vi "viewer0.1.vi"() -> ()   [LabVIEW 2020]
uses:
  <vilib>/Utility/file.llb/Read Delimited Spreadsheet (DBL).vi
panel:
  out "Intensity Graph 4":i32[][](graph)
  in  "Numeric":i32
  out "f":dbl=13.10591113674956
  out "t":dbl=0.07630144822178409
  in  "file path (dialog if empty)":path=path "W:/Labview/Front ends/ARPEScontrol/testfiles/1x1"
  out "Intensity Graph":dbl[][](graph)
  in  "e-size":u8=5
  in  "square thresh":i32=50
  in  "delta thresh":dbl=1.0
  in  "subtract":dbl=10.0
  # "4"
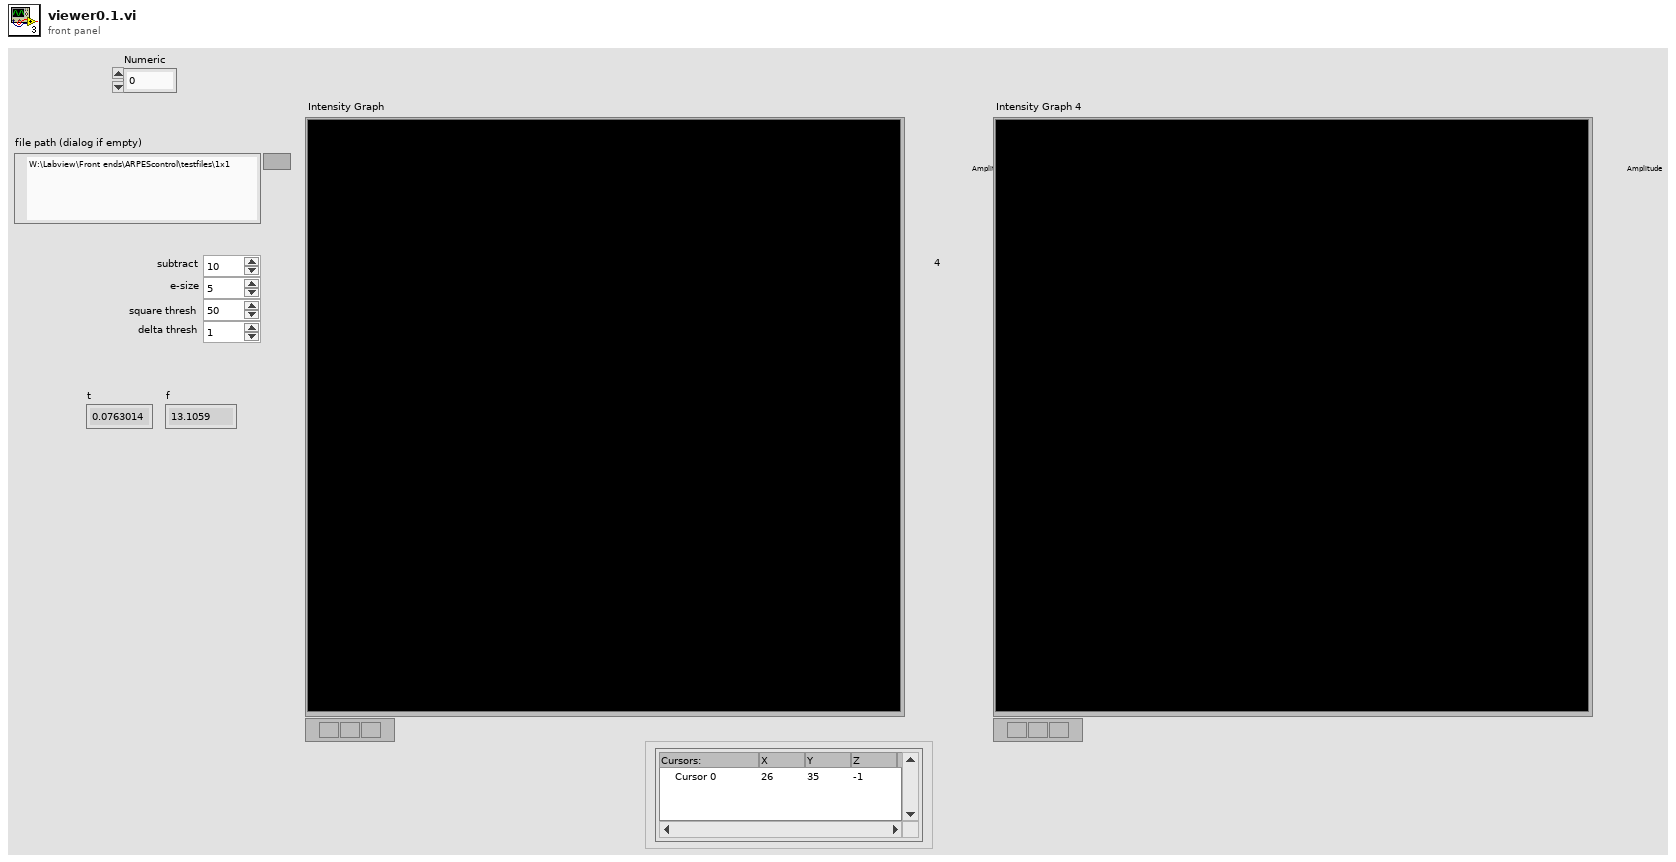
[diagram p1: front panel]
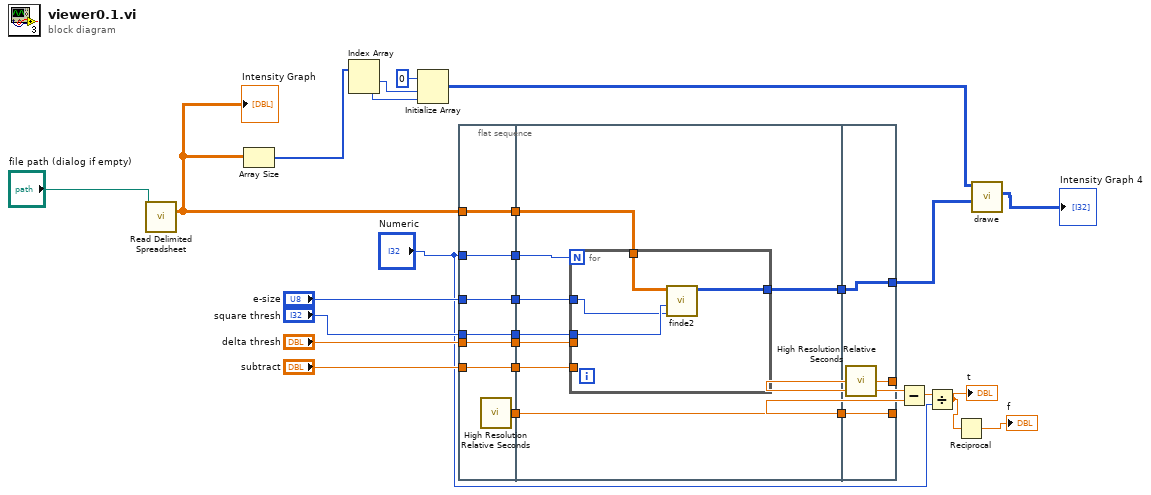
[diagram p0: block diagram]
diagram:
  n1 = call-poly <vilib>:"Read Delimited Spreadsheet.vi"("file path (dialog if empty)"="file path (dialog if empty)") -> ("all rows"=w24:dbl[][])  [unwired: 9 in, 5 out]
  "Intensity Graph" <- w24
  n2 = Array Size(array=w24) -> (size(s)=w23:i32[])
  n3 = Index Array(array=w23) -> (element #1=w22:i32, element #2=w21:i32)  [unwired: 2 in]
  n4 = Initialize Array(0 ("element"), w22, w21) -> (w4:i32[][])
  n5 = flat-sequence {
    tunnel: w24 -> [w31]
    tunnel: "e-size" -> [w32]
    tunnel: "square thresh" -> [w33]
    tunnel: "delta thresh" -> [w34]
    tunnel: "subtract" -> [w35]
    tunnel: [w35] -> w18
    tunnel: [w34] -> w17
    tunnel: [w33] -> w16
    tunnel: [w32] -> w15
    tunnel: [w31] -> w14
    tunnel: [w30] -> w13
    tunnel: [w29] -> w8
    tunnel: "Numeric" -> [w29]
    tunnel: w18 -> [w43]
    tunnel: w17 -> [w42]
    tunnel: w16 -> [w41]
    tunnel: w15 -> [w40]
    tunnel: w14 -> [w39]
    tunnel: w13 -> [w38]
    tunnel: [w38] -> w12
    tunnel: w8 -> [w37]
    tunnel: [w36] -> w1
    tunnel: w12 -> [w50]
    tunnel: [w50] -> w10
    tunnel: [w49] -> w11
    tunnel: [w48] -> w2
    tunnel: w1 -> [w48]
    frame #0 {
      n6 = call <vilib>:"High Resolution Relative Seconds.vi"() -> ("relative seconds"=w30:dbl)
    }
    frame #1 {
      n7 = for {
        N: w37 -> [_]
        tunnel: w43 -> [_]
        tunnel: w42 -> [_]
        tunnel: w41 -> [w46]
        tunnel: w40 -> [w45]
        tunnel: w39 -> [w47]
        tunnel: [w44] -> w36
        n8 = call "finde2.vi"("esize"=w45, "thresh"=w46, "inp array"=w47) -> ("locs"=w44:i32[][])  [unwired: 8 in]
      }
    }
    frame #2 {
      n9 = call <vilib>:"High Resolution Relative Seconds.vi"() -> ("relative seconds"=w49:dbl)
    }
  }
  n10 = Subtract(x=w11, y=w10) -> (x-y=w7:dbl)
  n11 = Divide(x=w7, y="Numeric") -> (x/y=w5:dbl)
  "t" <- w5
  n12 = Reciprocal(x=w5) -> (1/x=→"f":dbl)
  n13 = call "drawe.vi"("Xsize"=w2, "pos array"=w4) -> ("img out"=→"Intensity Graph 4":i32[][])  [unwired: 9 in]
